vi "applyLimit.vi"(8 "error in (no error)":errorcluster, 10 "Data":dbl[][](array[numeric]), 11 "HamegHMPSupply in":refnum<class "HamegHMPSupply.lvclass">) -> (0 "error out":errorcluster, 2 "Data":dbl[][](array[numeric]), 3 "HamegHMPSupply out":refnum<class "HamegHMPSupply.lvclass">)   [LabVIEW 2011, in "Hardware.lvlib" / "Channels.lvlib" / "HamegHMPSupply.lvclass"]
uses:
  HamegHMPSupply.lvclass
  AnalogOutput.lvclass
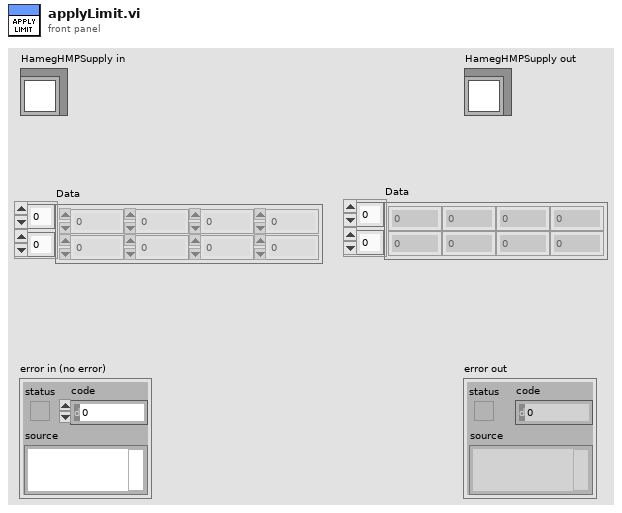
[diagram p1: front panel]
types:
  T1 = cluster{"VoltageLimit":dbl, "CurrentLimit":dbl}[]
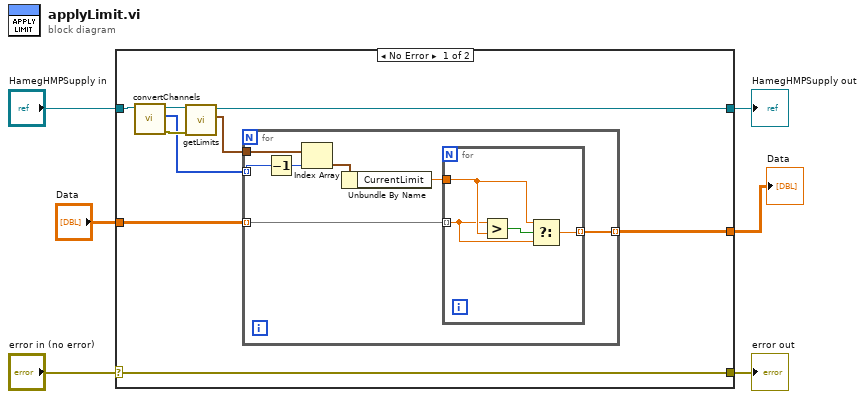
[diagram p0: block diagram]
diagram:
  n1 = case shown="No Error" "error in (no error)" {
    selector: "error in (no error)" -> [w15 w28]
    tunnel: [w15 w28] -> w5
    tunnel: [w13 w27] -> w3
    tunnel: "HamegHMPSupply in" -> [w11 w27]
    tunnel: "Data" -> [w14 _]
    tunnel: [w7 _] -> w1
    frame No Error {
      n2 = call "convertChannels.vi"("HamegHMPSupply in"=w11) -> ("error out"=w9:errorcluster, "channels"=w8:i32[], "HamegHMPSupply out"=w10:refnum<class "HamegHMPSupply.lvclass">)  [unwired: 8 in]
      n3 = call "getLimits.vi"("error in (no error)"=w9, "AnalogOutput in"=w10) -> ("Limits"=w12:T1, "AnalogOutput out"=w13:refnum<class "HamegHMPSupply.lvclass">)  [unwired: 7 in, 1 out]
      n4 = for {
        tunnel: w14 -> [w22] mode=indexing
        tunnel: w12 -> [w21]
        tunnel: w8 -> [w19] mode=indexing
        tunnel: [w16] -> w7 mode=indexing
        n5 = Decrement(x=w19) -> (x-1=w20:i32)
        n6 = Index Array(array=w21, index=w20) -> (element=w18:cluster{"VoltageLimit":dbl, "CurrentLimit":dbl})
        n7 = Unbundle By Name(w18) -> ("CurrentLimit"=w17:dbl)
        n8 = for {
          tunnel: w22 -> [w24] mode=indexing
          tunnel: w17 -> [w25]
          tunnel: [w23] -> w16 mode=indexing
          n9 = Greater?(x=w24, y=w25) -> (0:w26:bool)
          n10 = Select(t=w25, s=w26, f=w24) -> (s? t:f=w23:dbl)
        }
      }
    }
    frame Error {
    }
  }
  "error out" <- w5
  "HamegHMPSupply out" <- w3
  "Data" <- w1
